vi "FWCS_Communication.vi"() -> ()   [LabVIEW 2018]
uses:
  Stream/Stream.lvclass
  RxTx/RxTx.lvclass
  Stream/Stream.lvclass/Stream.ctl
panel:
  out "error out 2":errorcluster
  out "error out":errorcluster
  in  "RxTx.lvclass":refnum<class "RxTx.lvclass">
  in  "Stream.lvclass":refnum<class "Stream.lvclass">
  in  "RxTx.lvclass 2":refnum<class "RxTx.lvclass">
  in  "Stream.lvclass 2":refnum<class "Stream.lvclass">
  in  "Remote IP:":string="200.131.64.49"
  # "Filter Wheel Stream Communication"
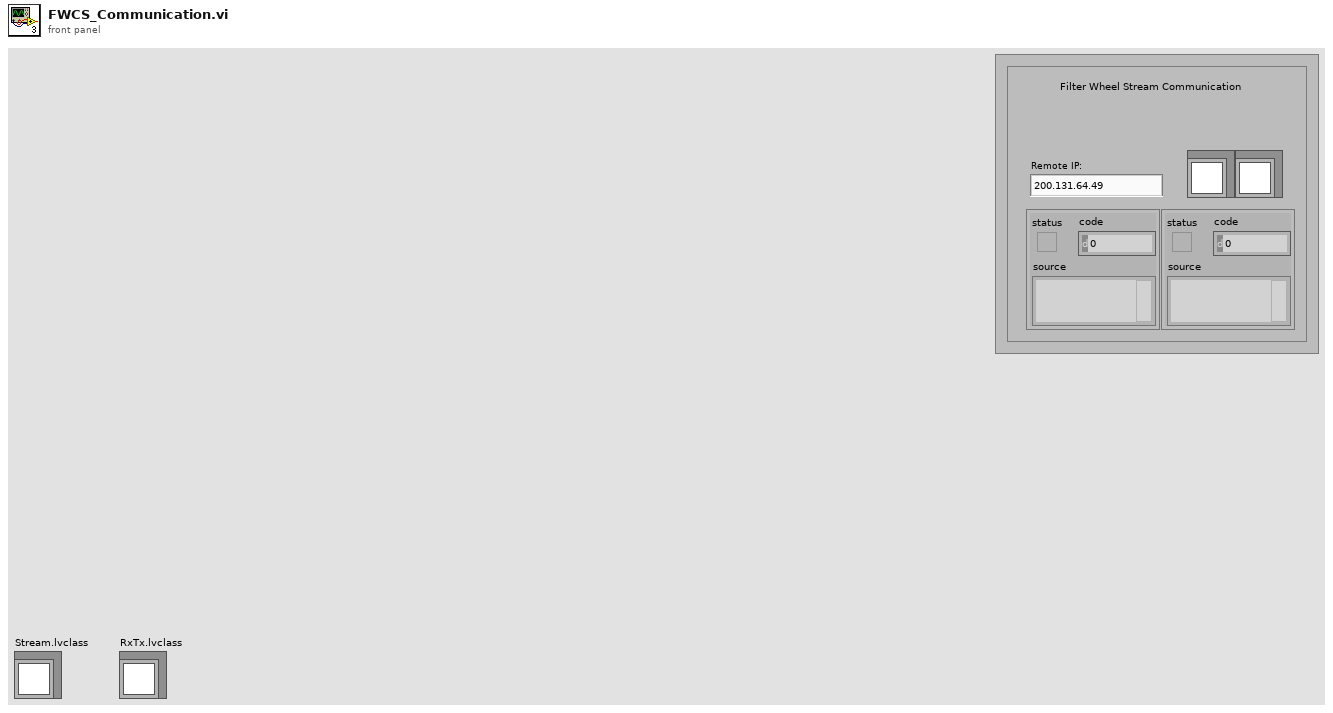
[diagram p1: front panel]
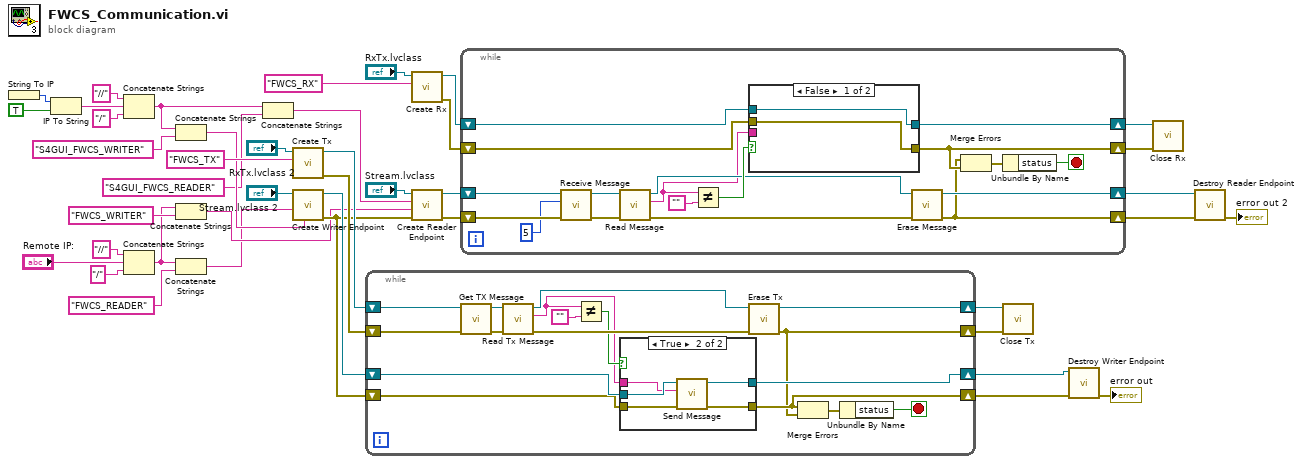
[diagram p0: block diagram]
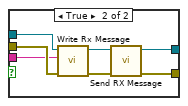
[diagram p2: hidden frame]
diagram:
  n1 = String To IP() -> (0:w15:u32)  [unwired: 1 in]
  n2 = IP To String(1:TRUE ("dot notation? (F)"), 2:w15) -> (0:w12:string)
  n3 = Concatenate Strings("//" ("Reader Name"), w12, "/" ("Reader Name")) -> (w9:string)
  n4 = Concatenate Strings("//" ("Reader Name"), "Remote IP:", "/" ("Reader Name")) -> (w3:string)
  n5 = Concatenate Strings(w9, "S4GUI_FWCS_WRITER" ("reader name")) -> (w30:string)
  n6 = Concatenate Strings(w3, "FWCS_WRITER" ("reader name")) -> (w6:string)
  n7 = Concatenate Strings(w3, "FWCS_READER" ("Reader Name")) -> (w5:string)
  n8 = Concatenate Strings(w9, "S4GUI_FWCS_READER" ("Reader Name")) -> (w21:string)
  n9 = call "Create Tx.vi"("Writer Name"="FWCS_TX" ("Reader Name"), "RxTx in"="RxTx.lvclass 2") -> ("error out"=w40:errorcluster, "RxTx out"=w41:refnum<class "RxTx.lvclass">)  [unwired: 8 in]
  n10 = call "Create Writer Endpoint.vi"("writer name"=w30, "reader name"=w5, "Stream in"="Stream.lvclass 2") -> ("error out"=w16:errorcluster, "Stream out"=w37:refnum<class "Stream.lvclass">)  [unwired: 7 in]
  n11 = while {
    shift-right: [w52] -> w35
    shift-left: w16 -> [w54]
    shift-right: [w53] -> w42
    shift-left: w37 -> [w55]
    shift-right: [w47] -> w38
    shift-left: w40 -> [w56]
    shift-right: [w49] -> w39
    shift-left: w41 -> [w57]
    stop <- w44 stop-if-true
    n12 = call "Get TX Message.vi"("error in (no error)"=w56, "RxTx in"=w57) -> ("error out"=w58:errorcluster, "RxTx out"=w45:refnum<class "RxTx.lvclass">)  [unwired: 8 in]
    n13 = call "Read Tx Message.vi"("error in (no error)"=w58, "RxTx in"=w45) -> ("error out"=w48:errorcluster, "Tx Message"=w43:string, "RxTx out"=w50:refnum<class "RxTx.lvclass">)  [unwired: 7 in]
    n14 = Not Equal?(x=w43, y="") -> (x != y?=w46:bool)
    n15 = case shown="True" w46 {
      tunnel: w55 -> [w61 w66]
      tunnel: w54 -> [w60 w65]
      tunnel: [w61 w64] -> w53
      tunnel: w43 -> [_ w63]
      tunnel: [w60 w62] -> w52
      frame False {
      }
      frame True {
        n16 = call "Send Message.vi"("error in (no error)"=w65, "Message"=w63, "Stream in"=w66) -> ("error out"=w62:errorcluster, "Stream out"=w64:refnum<class "Stream.lvclass">)  [unwired: 7 in]
      }
    }
    n17 = call "Erase Tx.vi"("error in (no error)"=w48, "RxTx in"=w50) -> ("error out"=w47:errorcluster, "RxTx out"=w49:refnum<class "RxTx.lvclass">)  [unwired: 8 in]
    n18 = Merge Errors(w52, w47) -> (w59:errorcluster)
    n19 = Unbundle By Name(w59) -> ("status"=w44:bool)
  }
  n20 = call "Create Rx.vi"("Reader Name"="FWCS_RX", "RxTx in"="RxTx.lvclass") -> ("error out"=w18:errorcluster, "RxTx out"=w19:refnum<class "RxTx.lvclass">)  [unwired: 8 in]
  n21 = call "Create Reader Endpoint.vi"("error in (no error)"=w16, "writer name"=w6, "reader name"=w21, "Stream in"="Stream.lvclass") -> ("error out"=w24:errorcluster, "Stream out"=w26:refnum<class "Stream.lvclass">)  [unwired: 6 in]
  n22 = while {
    shift-right: [w67] -> w23
    shift-left: w24 -> [w81]
    shift-right: [w70] -> w29
    shift-left: w26 -> [w82]
    shift-right: [w72] -> w27
    shift-left: w18 -> [w74]
    shift-right: [w73] -> w28
    shift-left: w19 -> [w75]
    stop <- w83 stop-if-true
    n23 = call "Receive Message.vi"("error in (no error)"=w81, "timeout ms"=5, "Stream in"=w82) -> ("error out"=w79:errorcluster, "Stream out"=w78:refnum<class "Stream.lvclass">)  [unwired: 7 in]
    n24 = call "Read Message.vi"("error in (no error)"=w79, "Stream in"=w78) -> ("error out"=w71:errorcluster, "Message"=w68:string, "Stream out"=w69:refnum<class "Stream.lvclass">)  [unwired: 7 in]
    n25 = Not Equal?(x=w68, y="") -> (x != y?=w77:bool)
    n26 = case shown="False" w77 {
      tunnel: w75 -> [w86 w93]
      tunnel: w74 -> [w85 w92]
      tunnel: [w86 w89] -> w73
      tunnel: [w85 w88] -> w72
      tunnel: w68 -> [_ w87]
      frame False {
      }
      frame True {
        n27 = call "Write Rx Message.vi"("error in (no error)"=w92, "Rx Message"=w87, "RxTx in"=w93) -> ("error out"=w91:errorcluster, "RxTx out"=w90:refnum<class "RxTx.lvclass">)  [unwired: 7 in]
        n28 = call "Send RX Message.vi"("error in (no error)"=w91, "RxTx in"=w90) -> ("error out"=w88:errorcluster, "RxTx out"=w89:refnum<class "RxTx.lvclass">)  [unwired: 8 in]
      }
    }
    n29 = call "Erase Message.vi"("error in (no error)"=w71, "Stream in"=w69) -> ("error out"=w67:errorcluster, "Stream out"=w70:refnum<class "Stream.lvclass">)  [unwired: 8 in]
    n30 = Merge Errors(w67, w72) -> (w84:errorcluster)
    n31 = Unbundle By Name(w84) -> ("status"=w83:bool)
  }
  n32 = call "Close Tx.vi"("error in (no error)"=w38, "RxTx in"=w39) -> ()  [unwired: 8 in, 2 out]
  n33 = call "Destroy Writer Endpoint.vi"("error in (no error)"=w35, "Stream in"=w42) -> ("error out"=→"error out":errorcluster)  [unwired: 8 in, 1 out]
  n34 = call "Close Rx.vi"("error in (no error)"=w27, "RxTx in"=w28) -> ()  [unwired: 8 in, 2 out]
  n35 = call "Destroy Reader Endpoint.vi"("error in (no error)"=w23, "Stream in"=w29) -> ("error out"=→"error out 2":errorcluster)  [unwired: 8 in, 1 out]
